vi "MinerRequestJob.vi"(3 "error in (no error)":errorcluster, 4 "UserName":string, 5 "connection ID":refnum<k5>) -> (0 "error out":errorcluster, 1 "job":string="2.4", 2 "connection ID out":refnum<k5>)   [LabVIEW 2014]
panel:
  out "error out 2":errorcluster
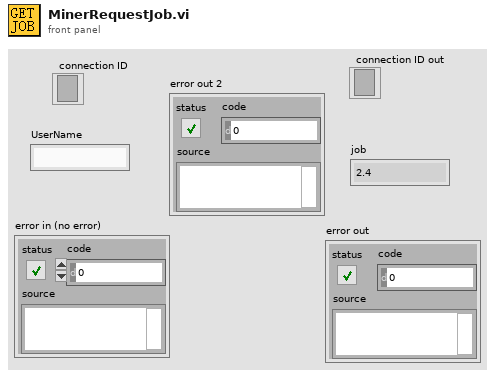
[diagram p1: front panel]
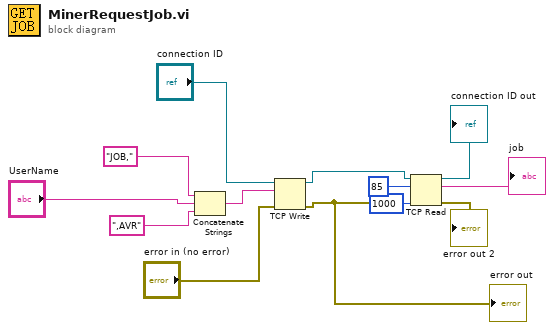
[diagram p0: block diagram]
diagram:
  n1 = Concatenate Strings("JOB," ("data in"), "UserName", ",AVR" ("data in")) -> (w9:string)
  n2 = TCP Write(connection ID="connection ID", data in=w9, error in (no error)="error in (no error)") -> (connection ID out=w6:refnum<k5>, error out=w2:errorcluster)  [unwired: 1 in, 1 out]
  "error out" <- w2
  n3 = TCP Read(connection ID=w6, bytes to read=85 ("读取的字节"), error in (no error)=w2, 9:1000 ("timeout ms (25000)")) -> (connection ID out=→"connection ID out":refnum<k5>, data out=→"job":string, error out=→"error out 2":errorcluster)  [unwired: 1 in]
